vi "SetTime.vi"(8 "error in (no error)":errorcluster, 10 "Time & Date":refnum<vi>, 11 "Init_T":bool) -> (0 "error out":errorcluster)   [LabVIEW 2017]
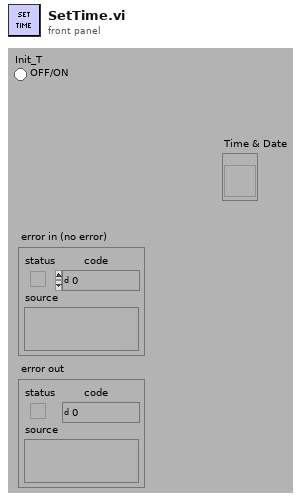
[diagram p1: front panel]
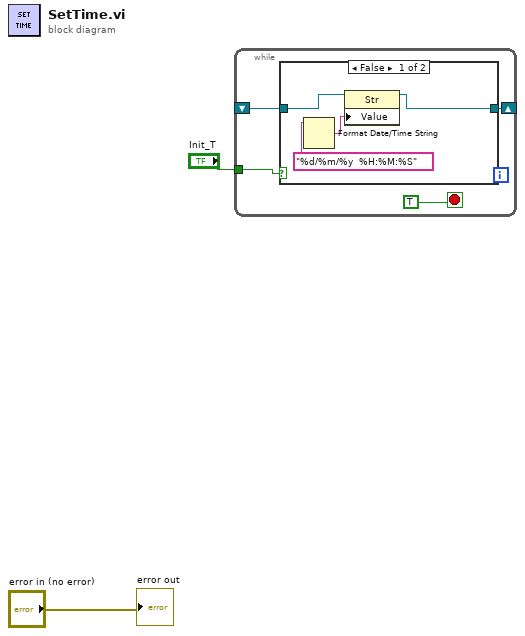
[diagram p0: block diagram]
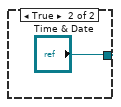
[diagram p2: hidden frame]
diagram:
  n1 = while {
    tunnel: "Init_T" -> [w5]
    shift-right: [w4] -> _
    shift-left: _ -> [w3]
    stop <- TRUE stop-if-true
    n2 = case shown="False" w5 {
      tunnel: [w9 "Time & Date"] -> w4
      tunnel: w3 -> [w10 _]
      frame False {
        n3 = Format Date/Time String(time format string (%c)="%d/%m/%y  %H:%M:%S") -> (date/time string=w8:string)  [unwired: 2 in]
        n4 = property class="Str"(reference=w10, "Value"=w8) -> (reference out=w9:refnum<vi>)  [unwired: 1 in, 1 out]
      }
      frame True {
      }
    }
  }
  "error out" <- "error in (no error)"
